vi "create 2D map act stats.vi"(8 "error in (no error)":errorcluster, 10 "Actuator array in":dbl[](array[numeric]), 11 "BMC in":refnum<class "BMC.lvclass">) -> (0 "error out":errorcluster, 2 "actuator stats out":dbl[][](array[numeric]), 3 "BMC out":refnum<class "BMC.lvclass">)   [LabVIEW 2012, in "BMC.lvclass"]
uses:
  BMC.lvclass
  BMC.lvclass/BMC.ctl
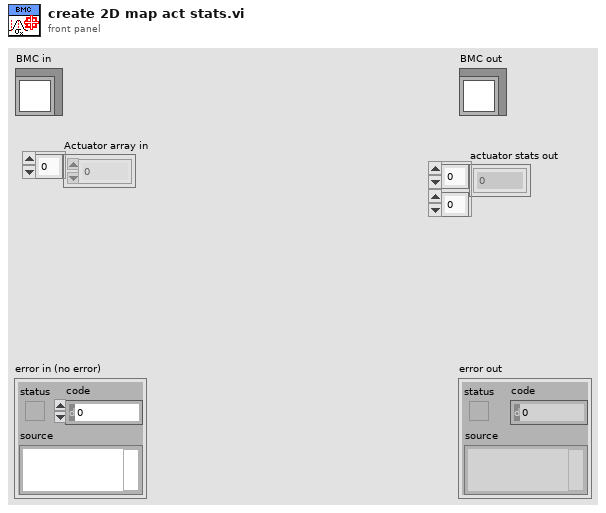
[diagram p1: front panel]
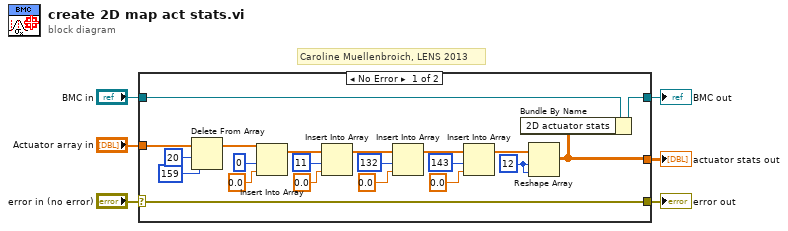
[diagram p0: block diagram]
diagram:
  # "Caroline Muellenbroich, LENS 2013"
  n1 = case shown="No Error" "error in (no error)" {
    selector: "error in (no error)" -> [w27 w29]
    tunnel: [w27 w29] -> w5
    tunnel: [w9 w28] -> w3
    tunnel: "BMC in" -> [w10 w28]
    tunnel: "Actuator array in" -> [w7 _]
    tunnel: [w8 _] -> w1
    frame No Error {
      w22 = 12 ("dimension size")
      n2 = Delete From Array(array=w7, length=20, index=159) -> (array with subset deleted=w26:dbl[])  [unwired: 1 out]
      n3 = Insert Into Array(array=w26, index=0, new element=0.0 ("new element/subarray")) -> (w15:dbl[])
      n4 = Insert Into Array(array=w15, index=11, new element=0.0 ("new element/subarray")) -> (w18:dbl[])
      n5 = Insert Into Array(array=w18, index=132, new element=0.0 ("new element/subarray")) -> (w21:dbl[])
      n6 = Insert Into Array(array=w21, index=143, new element=0.0 ("new element/subarray")) -> (w23:dbl[])
      n7 = Reshape Array(w23, w22, w22) -> (w8:dbl[][])
      n8 = Bundle By Name(cluster=w10, "2D actuator stats"=w8) -> (w9:refnum<class "BMC.lvclass">)
    }
    frame Error {
    }
  }
  "error out" <- w5
  "BMC out" <- w3
  "actuator stats out" <- w1
